vi "Ejemplo de examen.vi"() -> ()   [LabVIEW 2011]
panel:
  out "mayor>32":dbl
  out "Promedio Temp":dbl
  out "Mayor Temp":dbl
  out "Rango 31-50":bool
  out "Rango 21-30":bool
  out "Rango 1-20":bool
  out "Menor temp":dbl
  out "Temperatura":i32(slide) scale=0.0..50.0
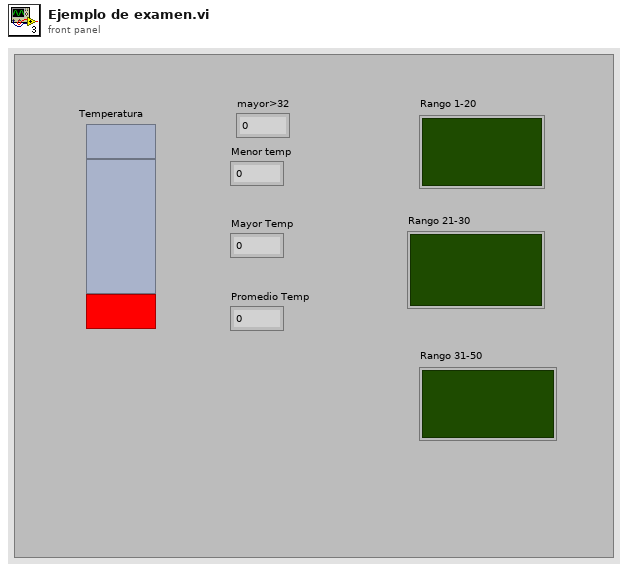
[diagram p1: front panel]
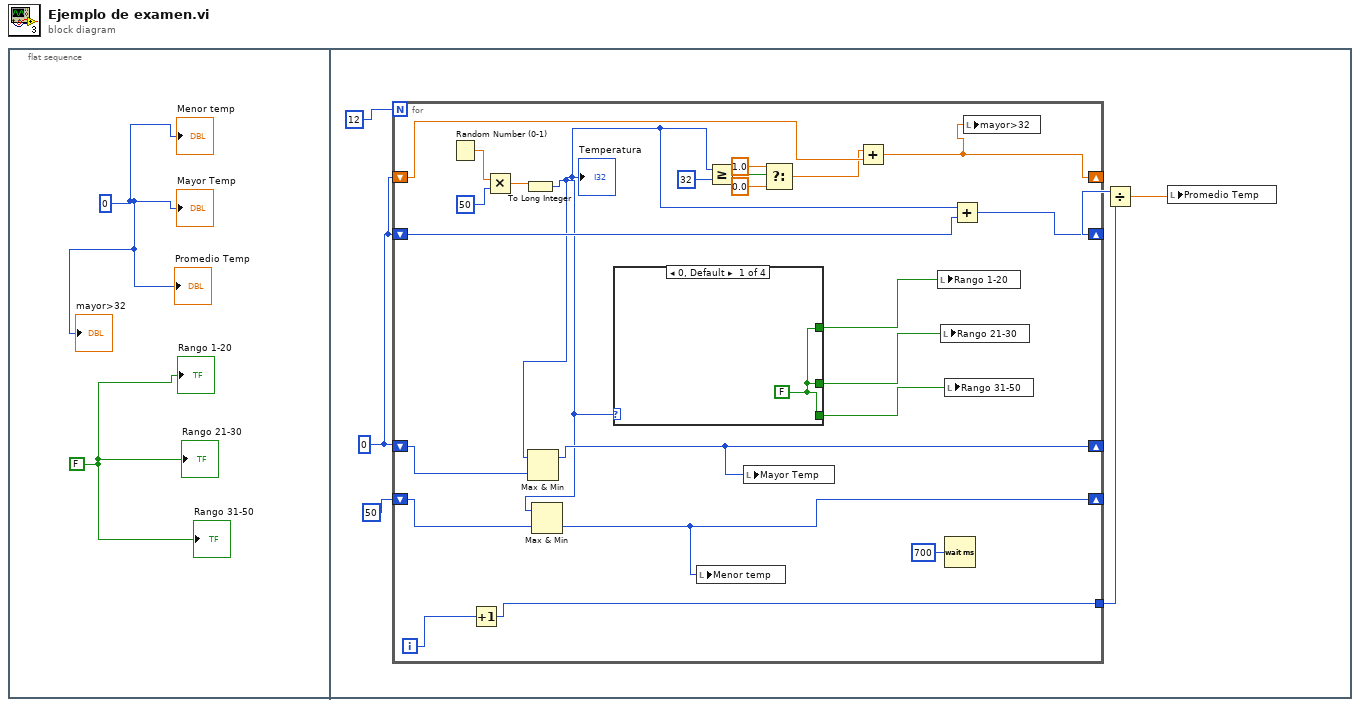
[diagram p0: block diagram]
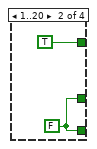
[diagram p2: hidden frame]
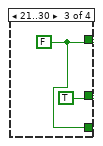
[diagram p3: hidden frame]
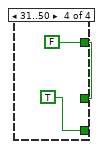
[diagram p4: hidden frame]
diagram:
  n1 = flat-sequence {
    frame #0 {
      w2 = FALSE
      w1 = 0
      "Menor temp" <- w1
      "Mayor Temp" <- w1
      "Promedio Temp" <- w1
      "Rango 1-20" <- w2
      "Rango 21-30" <- w2
      "Rango 31-50" <- w2
      "mayor>32" <- w1
    }
    frame #1 {
      w3 = 0
      n2 = for {
        N: 12 -> [_]
        shift-right: [w19] -> _
        shift-left: w3 -> [w20]
        shift-right: [w17] -> _
        shift-left: 50 -> [w18]
        shift-right: [w14] -> w6
        shift-left: w3 -> [w16]
        tunnel: [w12] -> w5
        shift-right: [w9] -> _
        shift-left: w3 -> [w11]
        i -> [w13]
        n3 = Random Number (0-1)() -> (number: 0 to 1=w31:dbl)
        n4 = Increment(x=w13) -> (x+1=w12:i32)
        n5 = Multiply(x=w31, y=50) -> (x*y=w29:dbl)
        n6 = To Long Integer(number=w29) -> (32bit integer=w15:i32)
        "Temperatura" <- w15
        n7 = Max & Min(x=w15, y=w20) -> (max(x,y)=w19:i32)  [unwired: 1 out]
        n8 = Max & Min(x=w15, y=w18) -> (min(x,y)=w17:i32)  [unwired: 1 out]
        n9 = case shown="0, Default" w15 {
          tunnel: [w32 TRUE w35 w37] -> w28
          tunnel: [w32 w33 TRUE w37] -> w27
          tunnel: [w32 w33 w35 TRUE] -> w26
          frame 0, Default {
            w32 = FALSE
          }
          frame 1..20 {
            w33 = FALSE
          }
          frame 21..30 {
            w35 = FALSE
          }
          frame 31..50 {
            w37 = FALSE
          }
        }
        n10 = local write "Menor temp"(w17) -> ()
        n11 = Greater Or Equal?(x=w15, y=32) -> (x >= y?=w24:bool)
        n12 = local write "Mayor Temp"(w19) -> ()
        n13 = Select(t=1.0, s=w24, f=0.0) -> (s? t:f=w10:dbl)
        n14 = Add(x=w10, y=w11) -> (x+y=w9:dbl)
        n15 = local write "Rango 1-20"(w28) -> ()
        n16 = local write "Rango 21-30"(w27) -> ()
        n17 = local write "Rango 31-50"(w26) -> ()
        n18 = Wait (ms)(milliseconds to wait=u32 700) -> ()  [unwired: 1 out]
        n19 = Add(x=w15, y=w16) -> (x+y=w14:i32)
        n20 = local write "mayor>32"(w9) -> ()
      }
      n21 = Divide(x=w6, y=w5) -> (x/y=w4:dbl)
      n22 = local write "Promedio Temp"(w4) -> ()
    }
  }
